vi "RT Loop - Log Data_4.vi"(8 "error in (no error)":errorcluster, 9 "Acceleration RT FIFO In":T1, 11 "Message Queue":refnum<queue>) -> ()   [LabVIEW 2017]
doc: "Receive triggered data from Analyze Acceleration Loop and log the data to disk."
uses:
  UI Error Handlers/support/Message Queue/Message Cluster.ctl
  controls/Acceleration RT FIFO Reference.ctl
  Globals/Global - All RT Loop Stop.vi
  Globals/Global - Configuration Options.vi
  UI Error Handlers/support/Logging/Logging.lvlib
  UI Error Handlers/support/Message Queue/Message Queue.lvlib
panel:
  out "error out":errorcluster
  out "Acceleration Log Folder":path=path "/home/lvuser/Log/logfiles_deploy"
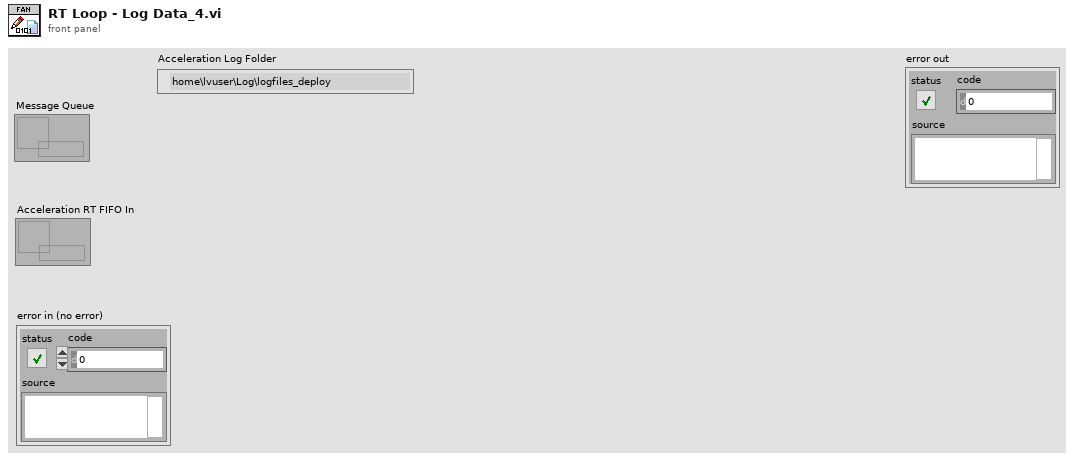
[diagram p1: front panel]
types:
  T1 = typedef "Acceleration RT FIFO Reference.ctl" = refnum<k33>
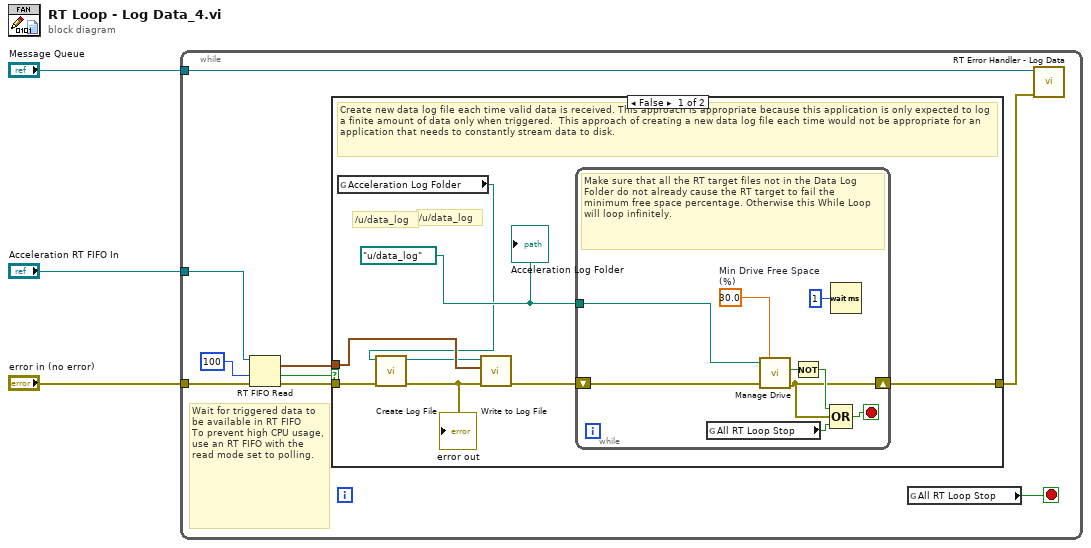
[diagram p0: block diagram]
diagram:
  n1 = while {
    tunnel: "Acceleration RT FIFO In" -> [w10]
    tunnel: "Message Queue" -> [w5]
    tunnel: "error in (no error)" -> [w12]
    stop <- w6 stop-if-true
    # "Wait for triggered data to be available in RT FIFO\nTo prevent high CPU usage, use an RT FIFO with the read mode set to polling."
    n2 = RT FIFO Read(0:w10, 2:100 ("ms timeout (0)"), 3:w12) -> (9:w7:waveform(dbl)[], 10:w8:bool, 11:w11:errorcluster)  [unwired: 1 in, 2 out]
    n3 = case shown="False" w8 {
      tunnel: w7 -> [w20 _]
      tunnel: w11 -> [w17 w30]
      tunnel: [w15 w30] -> w4
      frame False {
        w14 = path "u:/data_log" ("Acceleration Log Folder 2")
        # "/u/data_log"
        # "/u/data_log"
        # "Create new data log file each time valid data is received. This approach is appropriate because this application is only expected to log a finite amount of data only when triggered.  This approach of creating a new data log file each time would not be appropriate for an application that needs to constantly stream data to disk."
        n4 = global read "Global - Configuration Options.vi" "Acceleration Log Folder"() -> (w13:path)
        n5 = call "Create Log File.vi"("error in (no error)"=w17, "Acceleration Exceeded Log Folder"=w13) -> ("error out"=w18:errorcluster, "Log File out"=w16:refnum<k34>)  [unwired: 8 in]
        "error out" <- w18
        n6 = call "Write to Log File.vi"("error in (no error)"=w18, "Array of Waveforms"=w20, "Log File in"=w16) -> ("error out"=w19:errorcluster)  [unwired: 8 in]
        n7 = while {
          shift-right: [w24] -> w15
          shift-left: w19 -> [w25]
          tunnel: w14 -> [w22]
          stop <- w29 stop-if-true
          w23 = 30.0  # Min Drive Free Space (%)
          # "Make sure that all the RT target files not in the Data Log Folder do not already cause the RT target to fail the minimum free space percentage. Otherwise this While Loop will loop infinitely."
          n8 = global read "Global - All RT Loop Stop.vi" "All RT Loop Stop"() -> (w26:bool)
          n9 = call "Manage Drive.vi"("Min Drive Free Space (%)"=w23, "error in"=w25, "Data Folder"=w22) -> ("error out"=w24:errorcluster, "Drive Space Below Limit"=w21:bool)  [unwired: 6 in, 1 out]
          n10 = Not(x=w21) -> (.not. x?=w28:bool)
          n11 = Compound Arithmetic op=OR(w28, w24, w26) -> (w29:bool)
          n12 = Wait (ms)(milliseconds to wait=u32 1) -> ()  [unwired: 1 out]
        }
        "Acceleration Log Folder" <- w14
      }
      frame True {
        # "Timed out - No data"
      }
    }
    n13 = global read "Global - All RT Loop Stop.vi" "All RT Loop Stop"() -> (w6:bool)
    n14 = call "RT Error Handler - Log Data.vi"("error in (no error)"=w4, "Message Queue"=w5) -> ()  [unwired: 9 in, 1 out]
  }
